vi "PaneCoordsToScreenCoords.vi"(6 "VI":refnum<vi>, 8 "error in (no error)":errorcluster, 9 "Origin Pane":refnum<vi>, 10 "Owning Pane":refnum<vi>, 11 "Pane Coordinates":T1) -> (0 "error out":errorcluster, 3 "Screen Coords":T1)   [LabVIEW 2021, in "RocketPlot.lvlib"]
uses:
  RocketPlot.lvlib
  <vilib>/Utility/miscctls.llb/LVPointTypeDef.ctl
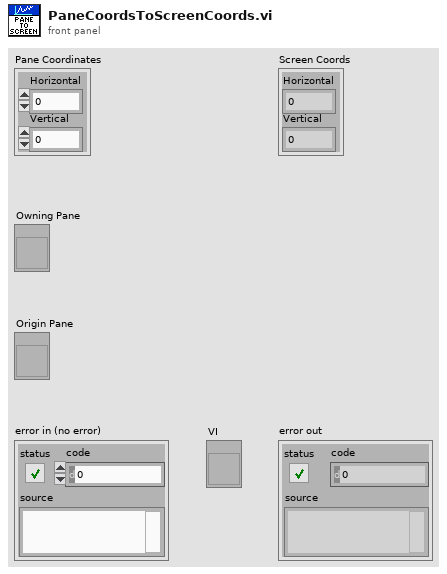
[diagram p1: front panel]
types:
  T1 = typedef "LVPointTypeDef.ctl" = cluster{"Horizontal":i16, "Vertical":i16}
  T2 = typedef "LVRectTypeDef.ctl" = cluster{"Left":i16, "Top":i16, "Right":i16, "Bottom":i16}
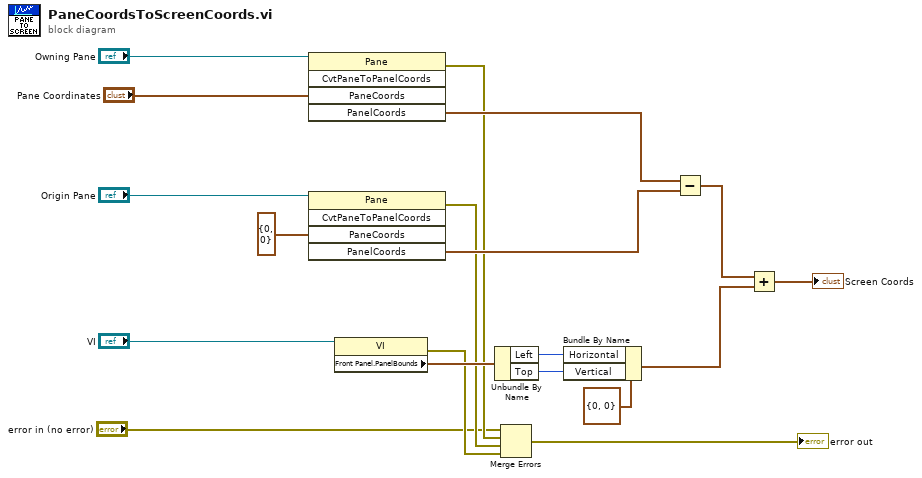
[diagram p0: block diagram]
diagram:
  n1 = invoke class="Pane" method="CvtPaneToPanelCoords"(reference="Owning Pane", "PaneCoords"="Pane Coordinates") -> (error out=w5:errorcluster, "PanelCoords"=w15:T1)  [unwired: 3 in, 3 out]
  n2 = invoke class="Pane" method="CvtPaneToPanelCoords"(reference="Origin Pane", "PaneCoords"=T1 {"Horizontal"=0, "Vertical"=0} ("Pane Coordinates")) -> (error out=w4:errorcluster, "PanelCoords"=w14:T1)  [unwired: 3 in, 3 out]
  n3 = property class="VI"(reference="VI") -> (error out=w3:errorcluster, "Front Panel.PanelBounds"=w13:T2)  [unwired: 1 in, 1 out]
  n4 = Unbundle By Name(w13) -> ("Left"=w11:i16, "Top"=w10:i16)
  n5 = Merge Errors("error in (no error)", w5, w4, w3) -> (→"error out":errorcluster)
  n6 = Bundle By Name(cluster=T1 {"Horizontal"=0, "Vertical"=0} ("Origin"), "Horizontal"=w11, "Vertical"=w10) -> (w8:T1)
  n7 = Subtract(x=w15, y=w14) -> (x-y=w9:T1)
  n8 = Add(x=w9, y=w8) -> (x+y=→"Screen Coords":T1)
